vi "asyncAcq_occRef_timeStamp_call.vi"(0 "spectrIdx":u16, 1 "channelIdx interferogram":u16, 2 "channelIdx spectrum":u16, 3 "FTSLV.dll path":path, 5 "error in (no error)":errorcluster, 6 "timeStamp interferogram":u32, 8 "timeStamp spectrum":u32) -> (10 "timeStamp spectrum latest":u32, 12 "timeStamp interferogram latest":u32, 13 "error":i32, 16 "new spectrum":bool, 18 "new interferogram":bool, 19 "error out":errorcluster)   [LabVIEW 2010, in "OSA.lvclass"]
doc: "SubVI to a <B>Thorlabs_OSA_64</B> object.\n\n[GOOP 1.0]"
uses:
  OSA.lvclass
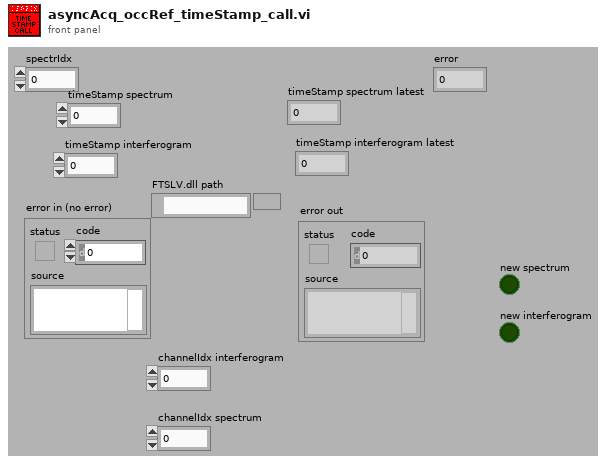
[diagram p1: front panel]
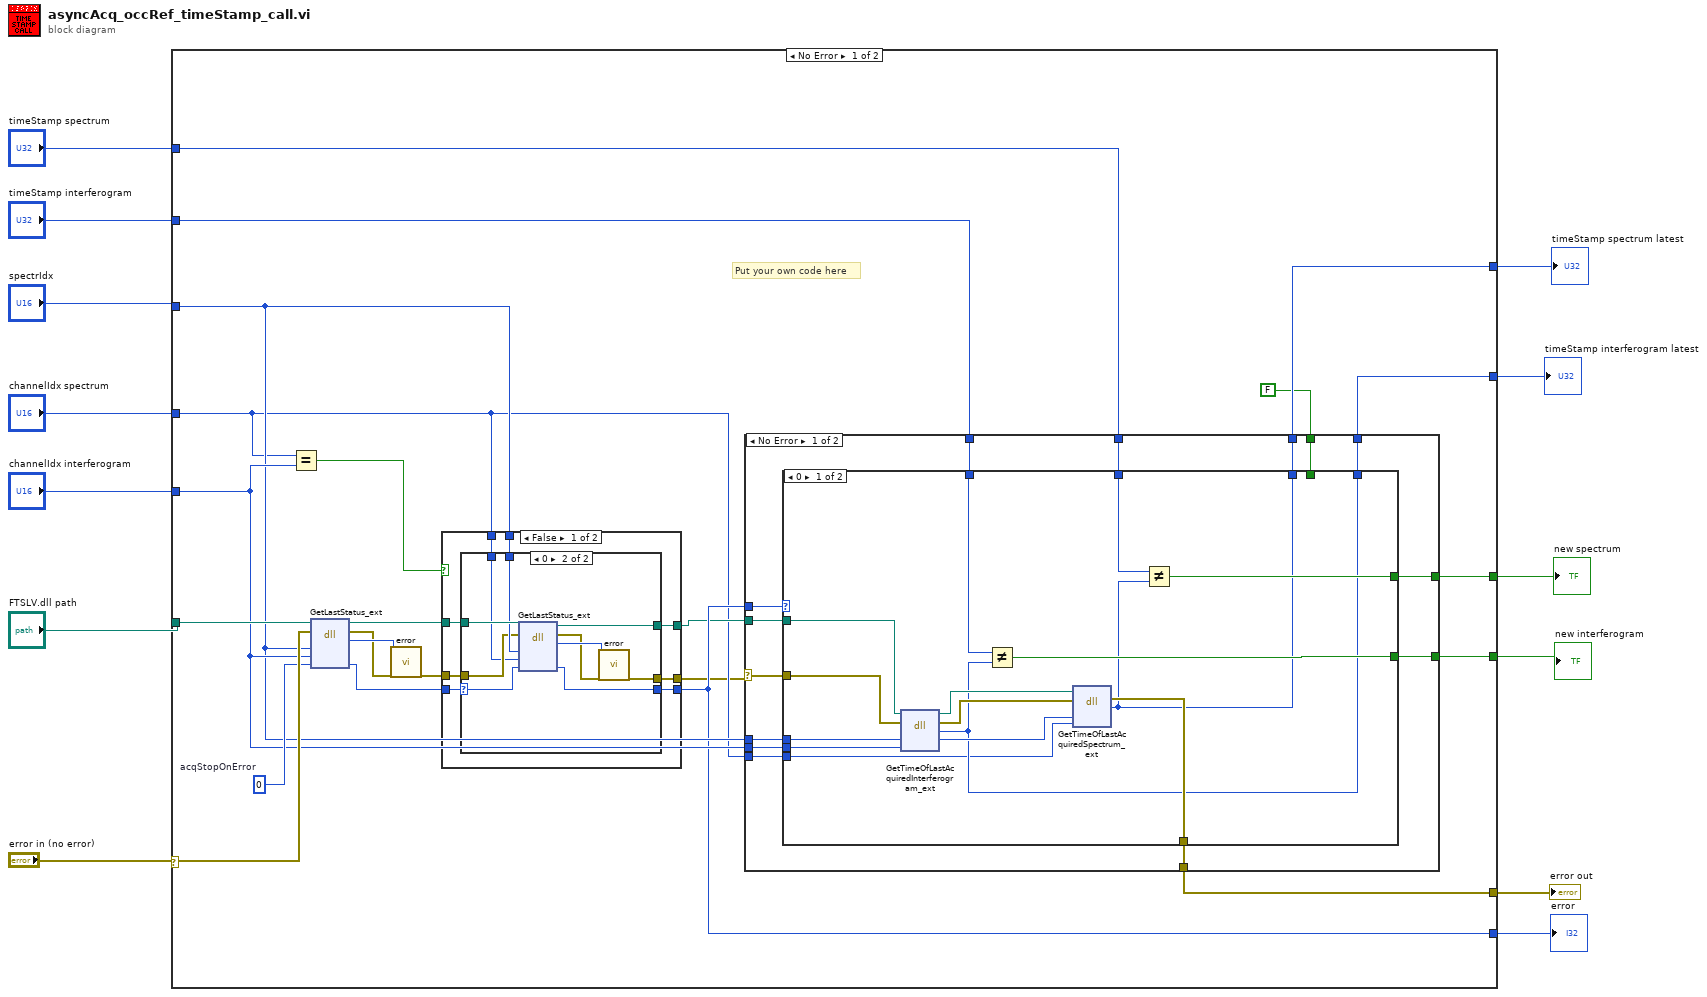
[diagram p0: block diagram]
diagram:
  n1 = case shown="No Error" "error in (no error)" {
    selector: "error in (no error)" -> [w30 w102]
    tunnel: [w27 w102] -> w13
    tunnel: "spectrIdx" -> [w18 _]
    tunnel: "timeStamp spectrum" -> [w36 w100]
    tunnel: "timeStamp interferogram" -> [w35 w101]
    tunnel: [w34 w100] -> w8
    tunnel: [w33 w101] -> w7
    tunnel: [w32 w99] -> w6
    tunnel: [w31 w99] -> w5
    tunnel: [w17 u8 0 ("acqStopOnError")] -> w4
    tunnel: "FTSLV.dll path" -> [w28 _]
    tunnel: "channelIdx interferogram" -> [w23 _]
    tunnel: "channelIdx spectrum" -> [w15 _]
    frame No Error {
      w26 = 0  # acqStopOnError
      # "Put your own code here"
      n2 = Equal?(x=w15, y=w23) -> (x = y?=w22:bool)
      n3 = dll-call lib="?" fn="GetLastStatus_ext" ("Thorlabs_FTS_asynchAcq.dll:Thorlabs_FTS_asynchAcq_handle")(path in=w28, error in=w30, "spectrIdx"=w18, "channel"=w23, "acqStopOnError"=w26) -> (path out=w19:path, error out=w24:errorcluster, "return type"=w25:u32, "acqStopOnError"=w21:i32)  [unwired: 3 in]
      n4 = call "error.vi"("result code"=w25, "error in (no error)"=w24) -> ("error out"=w20:errorcluster)  [unwired: 15 in, 2 out]
      n5 = case shown="False" w22 {
        tunnel: w21 -> [w44 w59]
        tunnel: w20 -> [w43 w58]
        tunnel: w19 -> [w42 w60]
        tunnel: [w41 w60] -> w16
        tunnel: w18 -> [w40 _]
        tunnel: w15 -> [w39 _]
        tunnel: [w38 w59] -> w17
        tunnel: [w37 w58] -> w14
        frame False {
          n6 = case shown="0" w44 {
            selector: w44 -> [w47 w50]
            tunnel: w43 -> [w45 w52]
            tunnel: w42 -> [w46 w55]
            tunnel: [w46 w54] -> w41
            tunnel: w40 -> [_ w53]
            tunnel: w39 -> [_ w51]
            tunnel: [w47 w49] -> w38
            tunnel: [w45 w48] -> w37
            frame Default {
            }
            frame 0 {
              n7 = dll-call lib="?" fn="GetLastStatus_ext" ("Thorlabs_FTS_asynchAcq.dll:Thorlabs_FTS_asynchAcq_handle")(path in=w55, error in=w52, "spectrIdx"=w53, "channel"=w51, "acqStopOnError"=w50) -> (path out=w54:path, error out=w56:errorcluster, "return type"=w57:u32, "acqStopOnError"=w49:i32)  [unwired: 3 in]
              n8 = call "error.vi"("result code"=w57, "error in (no error)"=w56) -> ("error out"=w48:errorcluster)  [unwired: 15 in, 2 out]
            }
          }
        }
        frame True {
        }
      }
      n9 = case shown="No Error" w14 {
        selector: w14 -> [w64 w94]
        tunnel: w18 -> [w74 _]
        tunnel: w36 -> [w73 w97]
        tunnel: w35 -> [w71 w96]
        tunnel: [w72 w95] -> w32
        tunnel: [w70 w95] -> w31
        tunnel: [w69 w97] -> w34
        tunnel: [w68 w96] -> w33
        tunnel: w17 -> [w67 _]
        tunnel: FALSE -> [w66 w95]
        tunnel: w16 -> [w65 _]
        tunnel: [w63 w94] -> w27
        tunnel: w23 -> [w62 _]
        tunnel: w15 -> [w61 _]
        frame No Error {
          n10 = case shown="0" w67 {
            tunnel: w74 -> [w89 _]
            tunnel: w73 -> [w83 w93]
            tunnel: [w81 w91] -> w72
            tunnel: w71 -> [w76 w92]
            tunnel: [w80 w91] -> w70
            tunnel: [w79 w93] -> w69
            tunnel: [w78 w92] -> w68
            tunnel: w66 -> [_ w91]
            tunnel: w65 -> [w87 _]
            tunnel: w64 -> [w85 w90]
            tunnel: [w82 w90] -> w63
            tunnel: w62 -> [w77 _]
            tunnel: w61 -> [w75 _]
            frame 0 {
              n11 = dll-call lib="?" fn="GetTimeOfLastAcquiredInterferogram_ext" ("Thorlabs_FTS_asynchAcq.dll:Thorlabs_FTS_asynchAcq_handle")(path in=w87, error in=w85, "spectrIdx"=w89, "channel"=w77) -> (path out=w86:path, error out=w84:errorcluster, "return type"=w78:u32, "spectrIdx"=w88:u16)  [unwired: 2 in]
              n12 = Not Equal?(x=w76, y=w78) -> (x != y?=w80:bool)
              n13 = dll-call lib="?" fn="GetTimeOfLastAcquiredSpectrum_ext" ("Thorlabs_FTS_asynchAcq.dll:Thorlabs_FTS_asynchAcq_handle")(path in=w86, error in=w84, "spectrIdx"=w88, "channel"=w75) -> (error out=w82:errorcluster, "return type"=w79:u32)  [unwired: 3 in, 1 out]
              n14 = Not Equal?(x=w83, y=w79) -> (x != y?=w81:bool)
            }
            frame Default {
            }
          }
        }
        frame Error {
        }
      }
    }
    frame Error {
      w99 = FALSE
      # "Error"
    }
  }
  "error out" <- w13
  "timeStamp interferogram latest" <- w7
  "timeStamp spectrum latest" <- w8
  "new spectrum" <- w6
  "new interferogram" <- w5
  "error" <- w4
